vi "getEventRejectedCommand.vi"(8 "error in (no error)":errorcluster, 11 "SALCommunicatorTC in":refnum<class "SALCommunicatorTC.lvclass">) -> (0 "error out":errorcluster, 1 "function return":i32, 2 "logevent_RejectedCommand_Ctl out":T1, 3 "SALCommunicatorTC out":refnum<class "SALCommunicatorTC.lvclass">)   [LabVIEW 2016, in "SALCommunicatorTC.lvclass"]
uses:
  SALCommunicatorTC/SALCommunicatorTC.lvclass
  ts_sallv_exa/DataTypes/logevent_RejectedCommand.ctl
  ts_sallv_exa/SALLV_EXA.lvlib
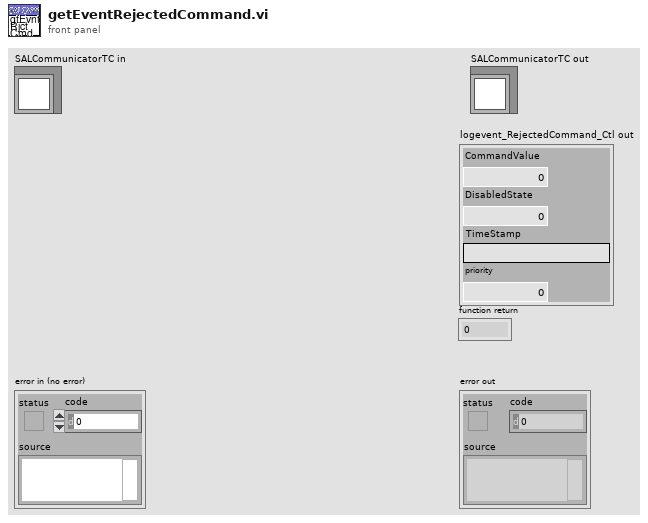
[diagram p1: front panel]
types:
  T1 = typedef "SALLV_EXA.lvlib/logevent_RejectedCommand.ctl" = cluster{"CommandValue":u16, "DisabledState":u16, "TimeStamp":string, "priority":i32}
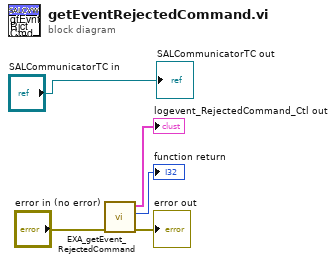
[diagram p0: block diagram]
diagram:
  n1 = call "EXA_getEvent_RejectedCommand.vi"("error in (no error)"="error in (no error)") -> ("error out"=→"error out":errorcluster, "function return"=→"function return":i32, "logevent_RejectedCommand_Ctl out"=→"logevent_RejectedCommand_Ctl out":T1)  [unwired: 8 in]
  "SALCommunicatorTC out" <- "SALCommunicatorTC in"
